vi "RT Loop - System Health and FPGA Monitoring.vi"(10 "FPGA VI Reference Out":T1, 11 "Message Queue":refnum<queue>) -> ()   [LabVIEW 2013]
uses:
  support/Message Queue/Message Cluster.ctl
  controls/FPGA VI Reference.ctl
  controls/FPGA State.ctl
  controls/Raw Values.ctl
  controls/Controller Calcs.ctl
  controls/Observer Calcs.ctl
  controls/Other Calcs.ctl
  Globals/Global - Configuration Options.vi
  <vilib>/nisyscfg/Close (System).vi
  Globals/Global - All RT Loop Stop.vi
  <vilib>/Utility/error.llb/Error Cluster From Error Code.vi
  <vilib>/rvi/errors/niLvFpgaAdjustHostInterfaceError.vi
  <vilib>/rvi/interface/nirviReadWriteControl/nirviReadWriteControl.xnode
  FPGA Bitfiles/crio-FPGA-contro_FPGATarget_FPGAMain_4HKUk4gb9wY.lvbitx
  <vilib>/NI_Real-Time Target Support.lvlib
  <vilib>/nisyscfg/nisyscfg.lvlib
  <resource>/objmgr/nisysapi.rc
  NiFpgaLv.dll
  support/Message Queue/Message Queue.lvlib
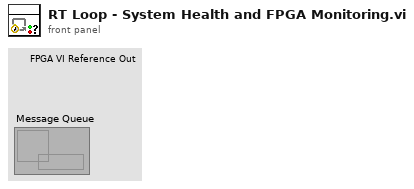
[diagram p1: front panel]
types:
  T1 = typedef "FPGA VI Reference.ctl" = refnum<k20>
  T2 = typedef "FPGA State.ctl" = enum16{"Safe State", "Manual", "Control (PID)"}
  T3 = typedef "Raw Values.ctl" = cluster{"Channel 0":fxp<+/-,20,7>, "Channel 1":fxp<+/-,20,7>, "Channel 2":fxp<+/-,20,7>, "Channel 3":fxp<+/-,20,14>}
  T4 = typedef "Controller Calcs.ctl" = cluster{"ba (kg/s)":fxp<+/-,20,7>, "ksa (N/m)":fxp<+/-,20,7>, "kisa (N/m)":fxp<+/-,20,7>, "k_backemf (Vs/m)":fxp<+/-,20,14>}
  T5 = typedef "Observer Calcs.ctl" = cluster{"bo (kg/s)":fxp<+/-,20,7>, "kso (N/m)":fxp<+/-,20,7>, "kiso (N/m)":fxp<+/-,20,7>}
  T6 = typedef "Other Calcs.ctl" = cluster{"k_1 (1/s)":fxp<+/-,20,7>, "k_2 (1/s)":fxp<+/-,20,7>, "Frr (N/s)":fxp<+/-,20,7>, "xrr (mm/s)":fxp<+/-,20,14>}
  T7 = typedef "NI_Real-Time Target Support.lvlib/RT CPU Load.ctl" = cluster{"Total (%)":dbl, "Time Critical (%)":dbl, "Timed Structures (%)":dbl, "High (%)":dbl, "Above Normal (%)":dbl, "Normal (%)":dbl, "Background (%)":dbl, "Idle (%)":dbl, "ISR (%)":dbl}
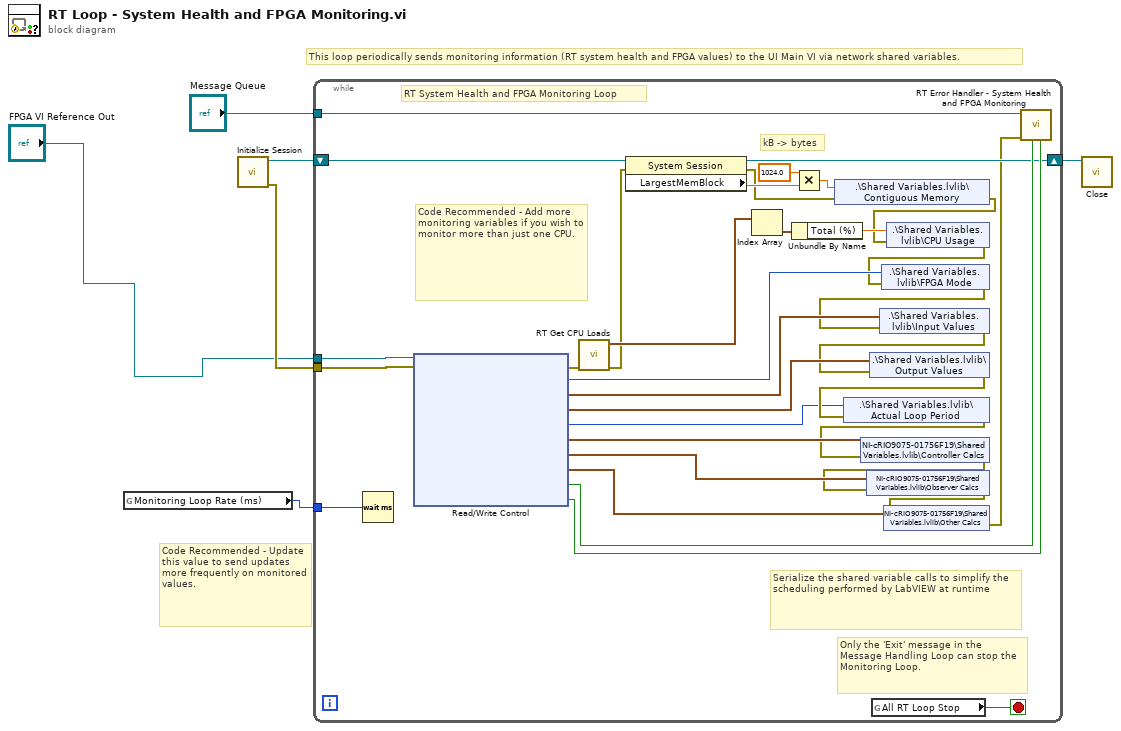
[diagram p0: block diagram]
diagram:
  # "Code Recommended - Update this value to send updates more frequently on monitored values."
  # "This loop periodically sends monitoring information (RT system health and FPGA values) to the UI Main VI via network shared variables."
  n1 = global read "Global - Configuration Options.vi" "Monitoring Loop Rate (ms)"() -> (w2:u32)
  n2 = call <vilib>:"Initialize Session.vi"() -> ("error out"=w3:errorcluster, "session out"=w5:refnum<k21>)  [unwired: 10 in]
  n3 = while {
    tunnel: "Message Queue" -> [w32]
    tunnel: "FPGA VI Reference Out" -> [w34]
    shift-right: [w19] -> w4
    shift-left: w5 -> [w23]
    tunnel: w3 -> [w16]
    tunnel: w2 -> [w14]
    stop <- w33 stop-if-true
    # "kB -> bytes"
    # "Serialize the shared variable calls to simplify the scheduling performed by LabVIEW at runtime"
    # "Code Recommended - Add more monitoring variables if you wish to monitor more than just one CPU."
    # "Only the 'Exit' message in the  Message Handling Loop can stop the Monitoring Loop."
    # "RT System Health and FPGA Monitoring Loop"
    n4 = Wait (ms)(milliseconds to wait=w14) -> ()  [unwired: 1 out]
    n5 = xnode "Read/Write Control"("FPGA VI Reference In"=w34, "error in"=w16) -> ("error out"=w29:errorcluster, "Current FPGA State"=w35:T2, "Input Values"=w36:T3, "Output Values"=w37:T3, "Actual Loop Period (ticks)"=w15:u32, "Controller Calcs"=w13:T4, "Observer Calcs"=w11:T5, "Other Calcs"=w9:T6, "Input Error"=w31:bool, "Output Error"=w30:bool)  [unwired: 1 out]
    n6 = call <vilib>:"RT Get CPU Loads.vi"("error in (no error)"=w29) -> ("error out"=w21:errorcluster, "CPU loads"=w40:T7[])  [unwired: 9 in]
    n7 = property class="System Session"(reference=w23, error in=w21) -> (reference out=w19:refnum<k21>, error out=w20:errorcluster, "LargestMemBlock"=w22:dbl)
    n8 = Index Array(array=w40) -> (element=w39:T7)  [unwired: 1 in]
    n9 = Unbundle By Name(w39) -> ("Total (%)"=w38:dbl)
    n10 = Multiply(x=1024.0, y=w22) -> (x*y=w18:dbl)
    n11 = shared-variable ".\\Shared Variables.lvlib\\Contiguous Memory"(w18, error in=w20) -> (error out=w25:errorcluster)
    n12 = global read "Global - All RT Loop Stop.vi" "All RT Loop Stop"() -> (w33:bool)
    n13 = shared-variable ".\\Shared Variables.lvlib\\CPU Usage"(w38, error in=w25) -> (error out=w24:errorcluster)
    n14 = shared-variable ".\\Shared Variables.lvlib\\FPGA Mode"(w35, error in=w24) -> (error out=w28:errorcluster)
    n15 = shared-variable ".\\Shared Variables.lvlib\\Input Values"(w36, error in=w28) -> (error out=w27:errorcluster)
    n16 = shared-variable ".\\Shared Variables.lvlib\\Output Values"(w37, error in=w27) -> (error out=w26:errorcluster)
    n17 = shared-variable ".\\Shared Variables.lvlib\\Actual Loop Period"(w15, error in=w26) -> (error out=w12:errorcluster)
    n18 = shared-variable "NI-cRIO9075-01756F19\\Shared Variables.lvlib\\Controller Calcs"(w13, error in=w12) -> (error out=w10:errorcluster)
    n19 = shared-variable "NI-cRIO9075-01756F19\\Shared Variables.lvlib\\Observer Calcs"(w11, error in=w10) -> (error out=w8:errorcluster)
    n20 = shared-variable "NI-cRIO9075-01756F19\\Shared Variables.lvlib\\Other Calcs"(w9, error in=w8) -> (error out=w7:errorcluster)
    n21 = call "RT Error Handler - System Health and FPGA Monitoring.vi"("Output Error (FPGA)"=w30, "Input Error (FPGA)"=w31, "error in (no error)"=w7, "Message Queue"=w32) -> ()  [unwired: 7 in, 1 out]
  }
  n22 = call-poly <vilib>:"Close.vi"("session in"=w4) -> ()  [unwired: 10 in, 1 out]
